vi "FileManager.vi"() -> ()   [LabVIEW 2019]
panel:
  in  "File index to get info":i32
  in  "File To Send":path caption="(Empty=No Action)"
  in  "To Folder":path caption="(Empty=No Action)"
  in  "File to Retrieve":string caption="(Empty=No Action)"
  out "# of Files":i32
  out "File info":T1
  out "File List":T2(array[cluster])
  out "FreeSpace":i32
  out "error out":errorcluster
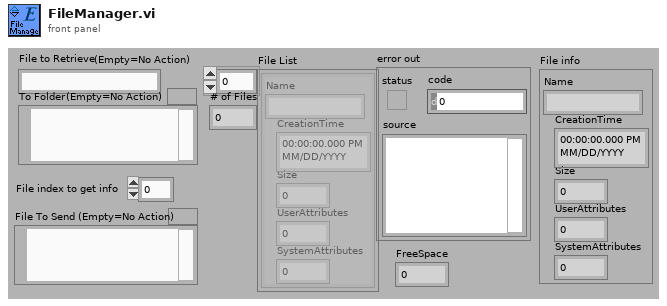
[diagram p1: front panel]
types:
  T1 = cluster{"Name":string, "CreationTime":timestamp, "Size":i32, "UserAttributes":i32, "SystemAttributes":i32}
  T2 = cluster{"Name":string, "CreationTime":timestamp, "Size":i32, "UserAttributes":i32, "SystemAttributes":i32}[]
  T3 = cluster{"Name":string, "CreationTime":timestamp, "Size":i32, "SystemAttributes":i32, "UserAttributes":i32}
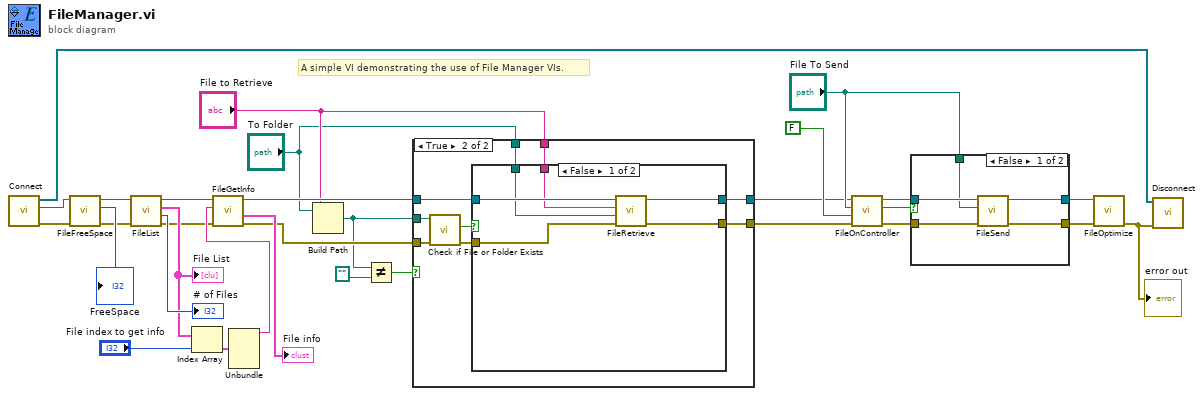
[diagram p0: block diagram]
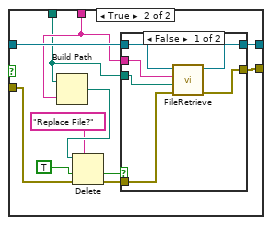
[diagram p3: hidden frame]
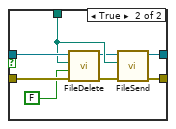
[diagram p5: hidden frame]
diagram:
  # "A simple VI demonstrating the use of File Manager VIs."
  n1 = call "Connect.vi"() -> ("error out"=w30:errorcluster, "controller"=w29:refnum<k24>, "controllers"=w31:refnum<k24>[])  [unwired: 9 in]
  n2 = call "FileFreeSpace.vi"("error in (no error)"=w30, "controller in"=w29) -> ("error out"=w26:errorcluster, "FreeSpace"=→"FreeSpace":i32, "controller out"=w27:refnum<k24>)  [unwired: 7 in]
  n3 = call "FileList.vi"("error in (no error)"=w26, "controller in"=w27) -> ("error out"=w11:errorcluster, "Number of Files"=→"# of Files":i32, "File List"=w15:T2, "controller out"=w10:refnum<k24>)  [unwired: 6 in]
  "File List" <- w15
  n4 = Index Array(array=w15, index="File index to get info") -> (element=w14:T1)
  n5 = Unbundle(w14) -> ("Name"=w13:string)  [unwired: 4 out]
  n6 = call "FileGetInfo.vi"("error in (no error)"=w11, "(Empty=No Action)"=w13, "controller in"=w10) -> ("error out"=w4:errorcluster, "File info Cluster"=→"File info":T3, "controller out"=w9:refnum<k24>)  [unwired: 6 in]
  n7 = Build Path(base path="To Folder", name or relative path="File to Retrieve") -> (appended path=w2:path)
  n8 = Not Equal?(x=w2, y=path "") -> (x != y?=w1:bool)
  n9 = case shown="True" w1 {
    tunnel: w9 -> [w33 w42]
    tunnel: [w33 w41] -> w8
    tunnel: [w32 w40] -> w7
    tunnel: "File to Retrieve" -> [_ w39]
    tunnel: "To Folder" -> [_ w38]
    tunnel: w4 -> [w32 w37]
    tunnel: w2 -> [_ w34]
    frame False {
      # "File does not exist, do not retrieve."
    }
    frame True {
      n10 = call <vilib>:"Check if File or Folder Exists.vi"("error in (no error)"=w37, "path"=w34) -> ("error out"=w36:errorcluster, "file or folder exists?"=w35:bool)  [unwired: 7 in, 1 out]
      n11 = case shown="False" w35 {
        tunnel: w42 -> [w48 w54]
        tunnel: [w47 w53] -> w41
        tunnel: w36 -> [w46 w58]
        tunnel: [w45 w55] -> w40
        tunnel: w39 -> [w44 w52]
        tunnel: w38 -> [w43 w51]
        frame False {
          n12 = call "FileRetrieve.vi"("error in (no error)"=w46, 9:"(Empty=No Action)"=w43, 10:"(Empty=No Action)"=w44, "controller in"=w48) -> ("error out"=w45:errorcluster, "controller out"=w47:refnum<k24>)  [unwired: 6 in]
        }
        frame True {
          n13 = Build Path(base path=w51, name or relative path=w52) -> (appended path=w59:path)
          n14 = Delete(prompt (Delete)="Replace File?" ("message"), path (use dialog)=w59, confirm (F)=TRUE, error in=w58) -> (cancelled=w57:bool, error out=w56:errorcluster)  [unwired: 1 in, 1 out]
          n15 = case shown="False" w57 {
            tunnel: w56 -> [w63 w67]
            tunnel: [w62 w67] -> w55
            tunnel: w54 -> [w65 w66]
            tunnel: [w64 w66] -> w53
            tunnel: w52 -> [w61 _]
            tunnel: w51 -> [w60 _]
            frame False {
              n16 = call "FileRetrieve.vi"("error in (no error)"=w63, 9:"(Empty=No Action)"=w60, 10:"(Empty=No Action)"=w61, "controller in"=w65) -> ("error out"=w62:errorcluster, "controller out"=w64:refnum<k24>)  [unwired: 6 in]
            }
            frame True {
            }
          }
        }
      }
    }
  }
  n17 = call "FileOnController.vi"("error in (no error)"=w7, "Silent?"=FALSE ("Notify?"), "(Empty=No Action)"="File To Send", "controller in"=w8) -> ("error out"=w23:errorcluster, "File Exist?"=w25:bool, "controller out"=w24:refnum<k24>)  [unwired: 5 in]
  n18 = case shown="False" w25 {
    tunnel: w24 -> [w72 w80]
    tunnel: [w71 w78] -> w22
    tunnel: w23 -> [w70 w79]
    tunnel: [w69 w77] -> w21
    tunnel: "File To Send" -> [w68 w76]
    frame False {
      n19 = call "FileSend.vi"("error in (no error)"=w70, "(Empty=No Action)"=w68, "controller in"=w72) -> ("error out"=w69:errorcluster, "controller out"=w71:refnum<k24>)  [unwired: 7 in]
    }
    frame True {
      n20 = call "FileDelete.vi"("error in (no error)"=w79, "Silent?"=FALSE, "(Empty=No Action)"=w76, "controller in"=w80) -> ("error out"=w75:errorcluster, "controller out"=w74:refnum<k24>)  [unwired: 6 in]
      n21 = call "FileSend.vi"("error in (no error)"=w75, "(Empty=No Action)"=w76, "controller in"=w74) -> ("error out"=w77:errorcluster, "controller out"=w78:refnum<k24>)  [unwired: 7 in]
    }
  }
  n22 = call "FileOptimize.vi"("error in (no error)"=w21, "controller in"=w22) -> ("error out"=w12:errorcluster)  [unwired: 8 in, 1 out]
  "error out" <- w12
  n23 = call "Disconnect.vi"("error in (no error)"=w12, "controllers"=w31) -> ()  [unwired: 9 in, 1 out]
